vi "Actor Core.vi"(8 "error in":errorcluster, 11 "Controller in":refnum<class "Controller.lvclass">) -> (0 "error out":errorcluster, 3 "Actor out":refnum<class "Actor.lvclass">)   [LabVIEW 2024, in "Controller.lvlib" / "Controller.lvclass"]
doc: "<p>(<strong>Filename</strong>: <span class=\"dnl\">Actor Framework.lvlib:Actor.lvclass:Actor Core.vi</span>)</p>\n<p>Receives messages to the actor, reacts to them, and initiates any error handling that may shut the actor down.</p>\n<p>Descendant classes may override this VI to append parallel tasks for the actor to complete while it handles messages. Overrides use the <a href=\"nihelplauncher://docs/csh?context=lvcore_glang_udclass\">Call Parent Class Method</a> node.</p>"
uses:
  Controller.lvclass
  C:/Program Files/National Instruments/LabVIEW 2024/vi.lib/ActorFramework/Actor/Actor.lvclass
  <vilib>/ActorFramework/Actor/Actor.lvclass
  MC Screen/MC Screen/Grid Screen.lvclass
  <vilib>/Utility/miscctls.llb/LVRectTypeDef.ctl
  Controller.lvclass/Controller.ctl
  <vilib>/ActorFramework/Actor/Actor.lvclass/Actor.ctl
  <vilib>/ActorFramework/Message Enqueuer/Message Enqueuer.lvclass/Message Enqueuer.ctl
  MC Screen/Grid Screen Messages/Assign Point Values to Grid Msg/Assign Point Values to Grid Msg.lvclass/Assign Point Values to Grid Msg.ctl
  47ef4eb2-3a5c-4d7f-8aa3-adaf7369ae0d.vi
  <vilib>/ActorFramework/Message Enqueuer/Init from Existing Queue.vi
  <vilib>/ActorFramework/Message Enqueuer/Enqueue.vi
  <vilib>/ActorFramework/Stop Msg/Stop Msg.lvclass
  C:/Program Files/National Instruments/LabVIEW 2024/vi.lib/ActorFramework/Message/Message.lvclass
  MC Screen/Grid Screen Messages/Assign Point Values to Grid Msg/Assign Point Values to Grid Msg.lvclass
  <vilib>/ActorFramework/Message Priority Queue/Priority Enqueue.vi
  <vilib>/ActorFramework/Message Enqueuer/Message Enqueuer.lvclass
  Controller Messages/Resize Image for Question Msg/Resize Image for Question Msg.lvclass
panel:
  out "Title":string="Challenge of the LabVIEW Champions!"
  out "String":string="TESTING TO SEE IF THIS LOOKS GOOD"
  out "Horizontal Graduated Bar":dbl(slide)=44.0 scale=0.0..100.0
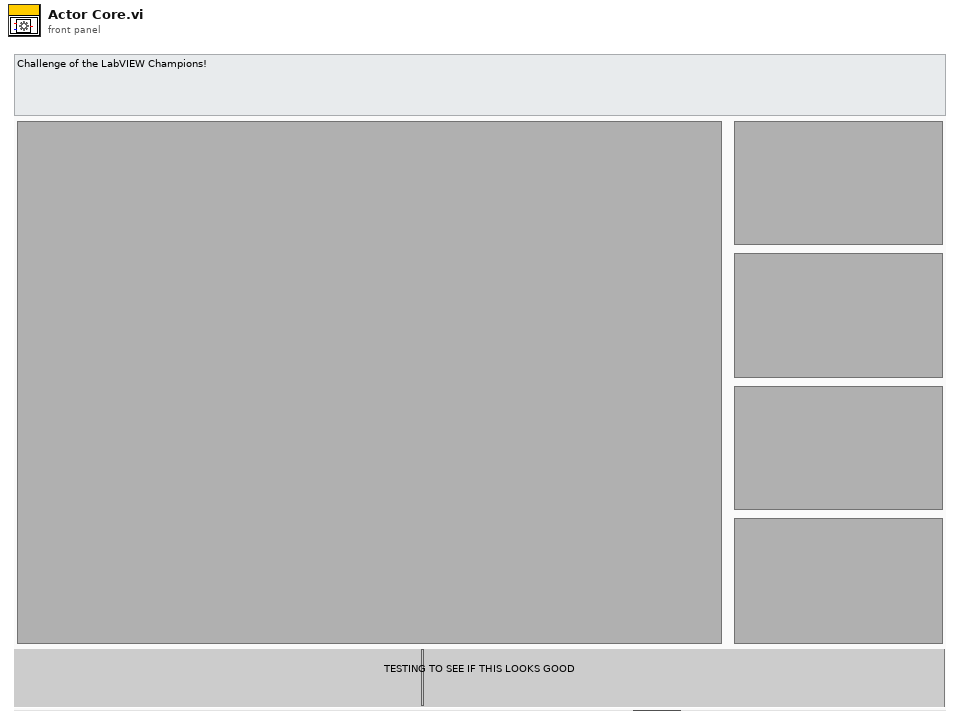
[diagram p1: front panel]
types:
  T1 = typedef "LVRectTypeDef.ctl" = cluster{"Left":i16, "Top":i16, "Right":i16, "Bottom":i16}
  T2 = enum16{"Sticks Top/Left", "Sticks Bottom/Right", "Proportional"}
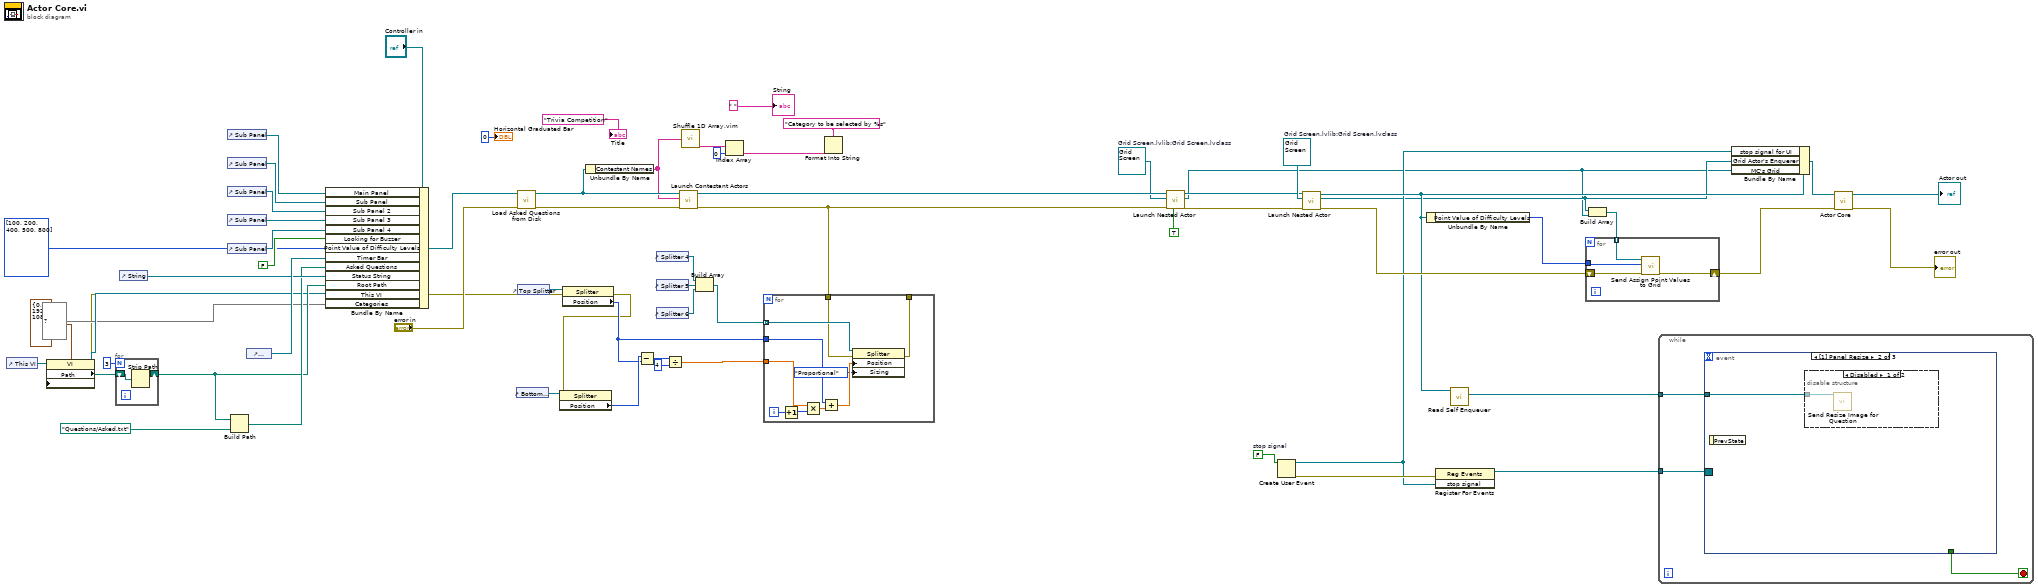
[diagram p0: block diagram]
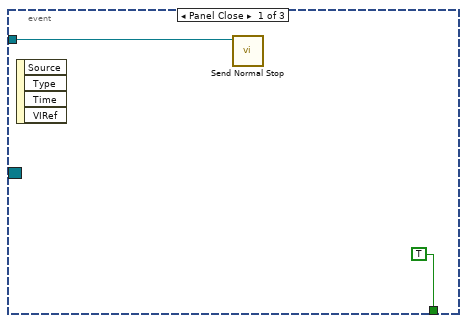
[diagram p2: hidden frame]
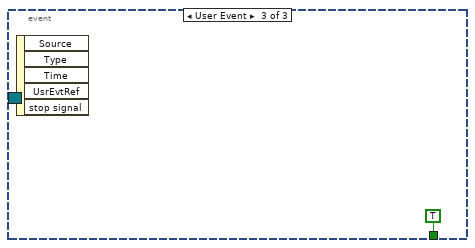
[diagram p4: hidden frame]
diagram:
  w9 = refnum<class "Grid Screen.lvclass"> refnum  # Grid Screen.lvlib:Grid Screen.lvclass
  w34 = FALSE  # stop signal
  w47 = refnum<class "Grid Screen.lvclass"> refnum  # Grid Screen.lvlib:Grid Screen.lvclass
  n1 = control-ref of="This VI"() -> (w21:refnum<vi>)
  n2 = property class="VI"(reference=w21, "Front Panel.WinBounds"=T1 {"Left"=0, "Top"=0, "Right"=1920, "Bottom"=1080} ("Front Panel Window:Window Bounds")) -> (reference out=w15:refnum<vi>, error out=w1:errorcluster, "Path"=w20:path)  [unwired: 1 in]
  n3 = for {
    N: 3 -> [_]
    shift-right: [w67] -> w16
    shift-left: w20 -> [w68]
    n4 = Strip Path(path=w68) -> (stripped path=w67:path)  [unwired: 1 out]
  }
  n5 = control-ref of="String"() -> (w24:refnum<vi>)
  n6 = control-ref of="Sub Panel"() -> (w52:refnum<vi>)
  n7 = control-ref of="Sub Panel"() -> (w51:refnum<vi>)
  n8 = control-ref of="Sub Panel"() -> (w50:refnum<vi>)
  n9 = control-ref of="Sub Panel"() -> (w49:refnum<vi>)
  n10 = control-ref of="Sub Panel"() -> (w48:refnum<vi>)
  n11 = Build Path(base path=w16, name or relative path=path "Questions/Asked.txt" ("Asked Questions")) -> (appended path=w17:path)
  n12 = control-ref of="Horizontal Graduated Bar"() -> (w41:refnum<vi>)
  n13 = Bundle By Name(cluster="Controller in", "Main Panel"=w52, "Sub Panel"=w51, "Sub Panel 2"=w50, "Sub Panel 3"=w49, "Sub Panel 4"=w48, "Looking for Buzzer"=FALSE, "Point Value of Difficulty Levels"=i32[] [100, 200, 400, 500, 800], "Timer Bar"=w41, "Asked Questions"=w17, "Status String"=w24, "Root Path"=w16, "This VI"=w15, "Categories"=set{string} {}) -> (w26:refnum<class "Controller.lvclass">)
  n14 = control-ref of="Bottom Splitter"() -> (w63:refnum<vi>)
  n15 = call-dynamic "Load Asked Questions from Disk.vi"("error in (no error)"="error in", "Controller in"=w26) -> ("error out"=w14:errorcluster, "Controller out"=w25:refnum<class "Controller.lvclass">)  [unwired: 8 in]
  n16 = control-ref of="Top Splitter"() -> (w64:refnum<vi>)
  n17 = property class="Splitter"(reference=w64, error in=w1) -> (error out=w2:errorcluster, "Position"=w54:i32)  [unwired: 1 out]
  n18 = property class="Splitter"(reference=w63, error in=w2) -> ("Position"=w62:i32)  [unwired: 2 out]
  n19 = Unbundle By Name(w25) -> ("Contestant Names"=w8:string[])
  n20 = Subtract(x=w62, y=w54) -> (x-y=w61:i32)
  n21 = control-ref of="Splitter 4"() -> (w57:refnum<vi>)
  n22 = control-ref of="Splitter 5"() -> (w58:refnum<vi>)
  n23 = control-ref of="Splitter 6"() -> (w59:refnum<vi>)
  n24 = Divide(x=w61, y=4) -> (x/y=w55:dbl)
  n25 = call "Launch Contestant Actors.vi"("error in (no error)"=w14, "Contestant Names"=w8, "Controller in"=w25) -> ("error out"=w53:errorcluster, "Controller out"=w22:refnum<class "Controller.lvclass">)  [unwired: 7 in]
  n26 = call "Shuffle 1D Array.vim"("array"=w8) -> ("shuffled array"=w6:string[])  [unwired: 4 in]
  n27 = Build Array(w57, w58, w59) -> (w56:refnum<vi>[])
  n28 = Index Array(array=w6, index=0) -> (element=w4:string)
  n29 = for {
    tunnel: w56 -> [w73] mode=indexing
    tunnel: w55 -> [w76]
    tunnel: w54 -> [w74]
    tunnel: [w70] -> _
    tunnel: w53 -> [w69]
    i -> [w78]
    n30 = Increment(x=w78) -> (x+1=w77:i32)
    n31 = Multiply(x=w76, y=w77) -> (x*y=w75:dbl)
    n32 = Add(x=w74, y=w75) -> (x+y=w72:dbl)
    n33 = property class="Splitter"(reference=w73, error in=w69, "Position"=w72, "Sizing"=T2."Proportional") -> (error out=w70:errorcluster)  [unwired: 1 out]
  }
  n34 = Format Into String(format string="Category to be selected by %s" ("initial string"), w4) -> ()  [unwired: 2 in, 2 out]
  n35 = call <vilib>:"Launch Nested Actor.vi"("Open Actor Core front panel? (F)"=TRUE, "error in (no error)"=w53, "Nested Actor"=w9, "Caller Actor in"=w22) -> ("error out"=w30:errorcluster, "Nested Actor's Enqueuer"=w28:refnum<class "Message Enqueuer.lvclass">, "Caller Actor out"=w31:refnum<class "Controller.lvclass">)  [unwired: 5 in]
  n36 = Create User Event(user event datatype=w34) -> (user event=w32:refnum<user-event>, error out=w35:errorcluster)  [unwired: 1 in]
  n37 = call <vilib>:"Launch Nested Actor.vi"("error in (no error)"=w30, "Nested Actor"=w47, "Caller Actor in"=w31) -> ("error out"=w39:errorcluster, "Nested Actor's Enqueuer"=w29:refnum<class "Message Enqueuer.lvclass">, "Caller Actor out"=w37:refnum<class "Controller.lvclass">)  [unwired: 6 in]
  n38 = Unbundle By Name(w37) -> ("Point Value of Difficulty Levels"=w43:i32[])
  n39 = register-events(error in=w35, w32) -> (reference out=w33:refnum<event-registration>)  [unwired: 1 in, 1 out]
  n40 = call <vilib>:"Read Self Enqueuer.vi"("Actor"=w37) -> ("Self Enqueuer"=w36:refnum<class "Message Enqueuer.lvclass">)  [unwired: 10 in]
  n41 = Build Array(w29, w28) -> (w27:refnum<class "Message Enqueuer.lvclass">[])
  n42 = for {
    tunnel: w27 -> [w82] mode=indexing
    tunnel: w43 -> [w81]
    shift-right: [w79] -> w38
    shift-left: w39 -> [w80]
    n43 = call "Send Assign Point Values to Grid.vi"("error in (no error)"=w80, "Point Value of Difficulty Levels"=w81, "Message Enqueuer"=w82) -> ("error out"=w79:errorcluster)  [unwired: 7 in, 1 out]
  }
  n44 = while {
    tunnel: w36 -> [w85]
    tunnel: w33 -> [w83]
    stop <- w84 stop-if-true
    n45 = event shown="[1] Panel Resize" {
      selector: w83 -> [_ _ _]
      dyn-events: _ -> [_ _ _]
      timeout: _ -> [_ _ _]
      tunnel: w85 -> [w87 w88 _]
      tunnel: [TRUE _ TRUE] -> w84
      event Panel Close {
        n46 = event-data() -> ()  [unwired: 1 in, 4 out]
        n47 = call <vilib>:"Send Normal Stop.vi"("Message Enqueuer"=w87) -> ()  [unwired: 10 in, 1 out]
      }
      event Panel Resize {
        n48 = event-data() -> ()  [unwired: 1 in, 1 out]
        n49 = disable-structure shown="Disabled" {
          disable-tunnel: w88 -> [w89 _]
          frame Disabled {
            n50 = call "Send Resize Image for Question.vi"("Message Enqueuer"=w89) -> ()  [unwired: 9 in, 2 out]
          }
          frame Enabled {
          }
        }
      }
      event User Event {
        n51 = event-data() -> ()  [unwired: 1 in, 5 out]
      }
    }
  }
  n52 = Bundle By Name(cluster=w37, "stop signal for UI"=w32, "Grid Actor's Enquerer"=w29, "MC's Grid"=w28) -> (w46:refnum<class "Controller.lvclass">)
  n53 = call-parent "Actor Core.vi"("error in"=w38, "Actor in"=w46) -> ("error out"=→"error out":errorcluster, "Actor out"=→"Actor out":refnum<class "Actor.lvclass">)  [unwired: 8 in]
  "Title" <- "Trivia Competition" ("Title")
  "Horizontal Graduated Bar" <- u8 0 ("Horizontal Graduated Bar")
  "String" <- " " ("String")
